vi "GDSString_ParseDataTypeString.vi"(10 "DefaultAccessScope(Private)":T1, 11 "InputText":string) -> (1 "DataTypeString":string, 2 "Found":bool, 3 "DataType":T2)   [LabVIEW 2012]
uses:
  <resource>/Framework/Providers/Open_GDS/ClassProviders/Common/CommonVIs/CommonVIs_AttributeType.ctl
  <resource>/Framework/Providers/Open_GDS/ClassProviders/Common/CommonVIs/CommonVIs_AttributeDataType.ctl
  <resource>/Framework/Providers/Open_GDS/ClassProviders/Common/String/GDSString_AccessScopeModifierType.ctl
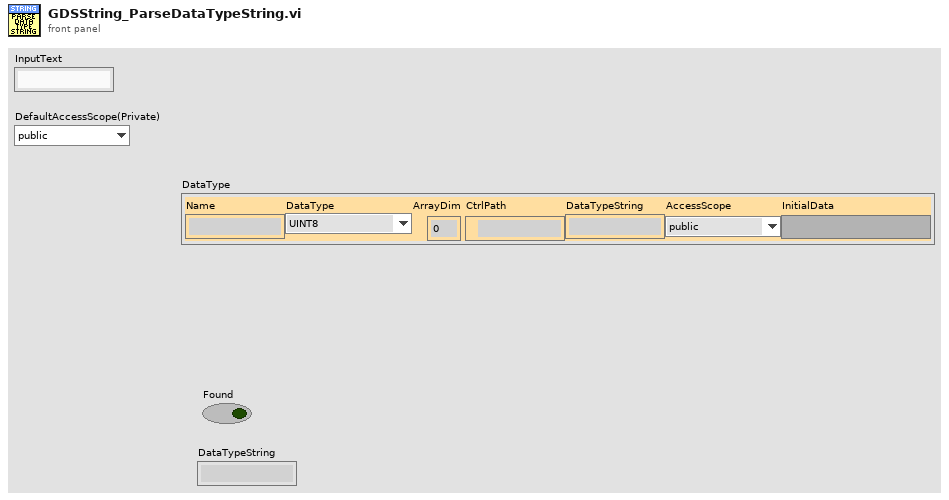
[diagram p1: front panel]
types:
  T1 = typedef "GDSString_AccessScopeModifierType.ctl" = enum16{"public", "private", "protected", "internal"}
  T2 = typedef "CommonVIs_AttributeType.ctl" = cluster{"Name":string, "DataType":T3, "ArrayDim":i32, "CtrlPath":path, "DataTypeString":string, "AccessScope":T1, "InitialData":variant}
  T3 = typedef "CommonVIs_AttributeDataType.ctl" = enum16{"UINT8", "INT8", "UINT16", "INT16", "UINT32", "INT32", "UINT64", "INT64", "SGL", "DBL", "EXT", "CSG", "CDB", "CXT", "TimeStamp", "STRING", "PATH", "BOOL", "ENUM", "RefNum", "VIRefNum", "LabVIEW Class", "Cluster", "Variant", "TypeDef", "Waveform", "LabVIEW Object", "Other", "void"}
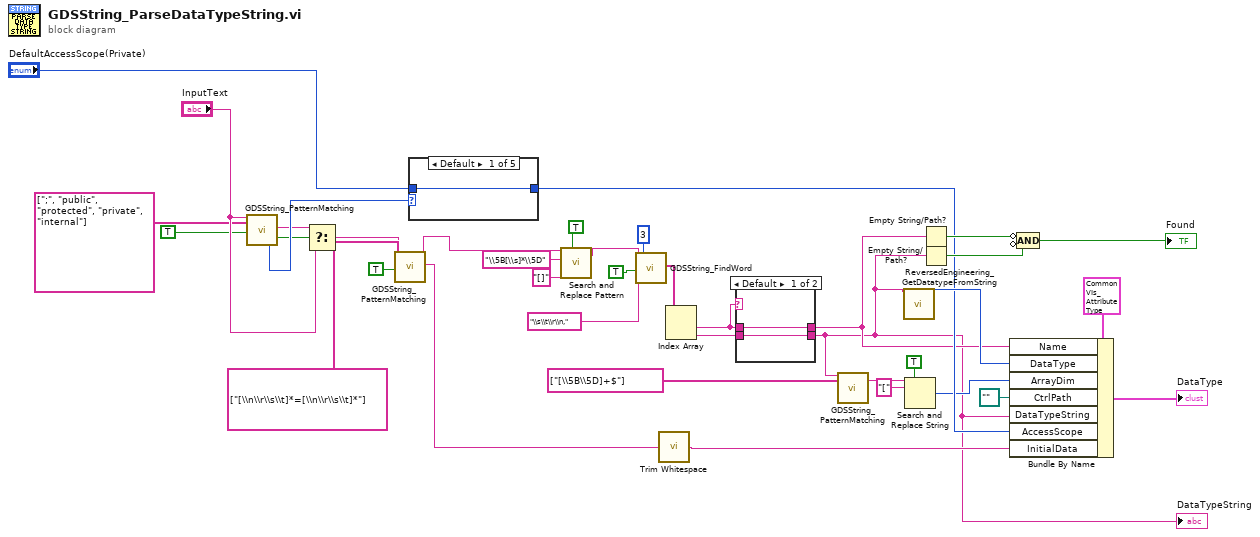
[diagram p0: block diagram]
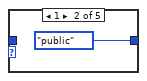
[diagram p3: hidden frame]
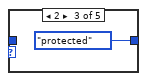
[diagram p4: hidden frame]
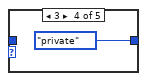
[diagram p5: hidden frame]
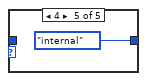
[diagram p6: hidden frame]
diagram:
  n1 = call <resource>:"GDSString_PatternMatching.vi"("TextIn"="InputText", "PatternMatchingStrings"=string[] [";", "public", "protected", "private", "internal"] ("PatternMatchingString"), "Search Backwards"=TRUE) -> ("IndexOfTheFoundPatternMatchingString"=w16:i32, "TextAfter"=w9:string, "Found"=w8:bool)  [unwired: 10 in, 4 out]
  n2 = Select(t=w9, s=w8, f="InputText") -> (s? t:f=w11:string)
  n3 = call <resource>:"GDSString_PatternMatching.vi"("TextIn"=w11, "PatternMatchingStrings"=string[] ["[\\n\\r\\s\\t]*=[\\n\\r\\s\\t]*"] ("PatternMatchingString"), "Search Backwards"=TRUE) -> ("TextBefore"=w30:string, "TextAfter"=w24:string)  [unwired: 10 in, 5 out]
  n4 = case shown="Default" w16 {
    tunnel: [w39 GDSString_AccessScopeModifierType."public" ("AccessScope") GDSString_AccessScopeModifierType."protected" ("AccessScope") GDSString_AccessScopeModifierType."private" ("AccessScope") GDSString_AccessScopeModifierType."internal" ("AccessScope")] -> w23
    tunnel: "DefaultAccessScope(Private)" -> [w39 _ _ _ _]
    frame Default {
    }
    frame 1 {
    }
    frame 2 {
    }
    frame 3 {
    }
    frame 4 {
    }
  }
  n5 = call <vilib>:"Search and Replace Pattern.vi"("string"=w30, "regular expression (\"\")"="\\5B[\\s]*\\5D" ("regular expression (\"\")"), "replace string (\"\")"="[]" ("replace string (\"\")"), "replace all? (F)"=TRUE) -> ("result string"=w31:string)  [unwired: 1 in, 1 out]
  n6 = call <resource>:"GDSString_FindWord.vi"("Text"=w31, "PatternMatchingDelimiter(\\s\\t\\r\\n)"="\\s\\t\\r\\n," ("PatternMatchingDelimiter(\\s\\t\\r\\n)"), "Search Backwards"=TRUE, "GetNext-X_Words(1,-1=All)"=3) -> ("NextWords"=w18:string[])  [unwired: 10 in, 5 out]
  n7 = call <vilib>:"Trim Whitespace.vi"("string"=w24) -> ("trimmed string"=w25:string)  [unwired: 1 in]
  n8 = Index Array(array=w18) -> (element #1=w5:string, element #2=w3:string)  [unwired: 2 in]
  n9 = case shown="Default" w5 {
    tunnel: [w45 w46] -> w4
    tunnel: w5 -> [w45 w46]
    tunnel: [w44 w46] -> w2
    tunnel: w3 -> [w44 _]
    frame Default {
    }
    frame "void" {
    }
  }
  "DataTypeString" <- w2
  n10 = call <resource>:"GDSString_PatternMatching.vi"("TextIn"=w2, "PatternMatchingStrings"=string[] ["[\\5B\\5D]+$"] ("PatternMatchingString")) -> ("Match"=w20:string)  [unwired: 11 in, 6 out]
  n11 = call <resource>:"ReversedEngineering_GetDatatypeFromString.vi"("String"=w2) -> ("AttributeDataType"=w38:T3)  [unwired: 10 in, 4 out]
  n12 = Search and Replace String(replace all?=TRUE ("replace all? (F)"), input string=w20, search string="[") -> (number of replacements=w22:i32)  [unwired: 5 in, 3 out]
  n13 = Empty String/Path?(string/path=w4) -> (empty?=w27:bool)
  n14 = Empty String/Path?(string/path=w2) -> (empty?=w28:bool)
  n15 = Bundle By Name(cluster=T2 {"Name"="", "DataType"=enum."UINT8", "ArrayDim"=0, "CtrlPath"=path "", "DataTypeString"="", "AccessScope"=enum."public", "InitialData"=variant} ("DataType"), "Name"=w4, "DataType"=w38, "ArrayDim"=w22, "CtrlPath"=path "", "DataTypeString"=w2, "AccessScope"=w23, "InitialData"=w25) -> (→"DataType":T2)
  n16 = Compound Arithmetic op=AND(invert w27, invert w28) -> (→"Found":bool)
